vi "mainObjectivesRegistration.vi"() -> ()   [LabVIEW 2017]
uses:
  globalUtilities.vi
  globalDevices.vi
  <userlib>/Hamamatsu Video Capture/tm_getframe16_40.vi
  <vilib>/Analysis/baseanly.llb/Std Deviation and Variance.vi
  <vilib>/Analysis/NI_AALPro.lvlib
panel:
  in  "galvo N-1 2":i32
  in  "piezo M 2":i32=1
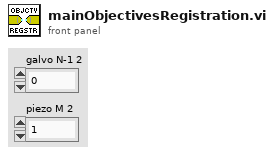
[diagram p1: front panel]
types:
  T1 = cluster{"initial amplitude":dbl, "initial center":dbl, "initial standard deviation":dbl, "offset":dbl}
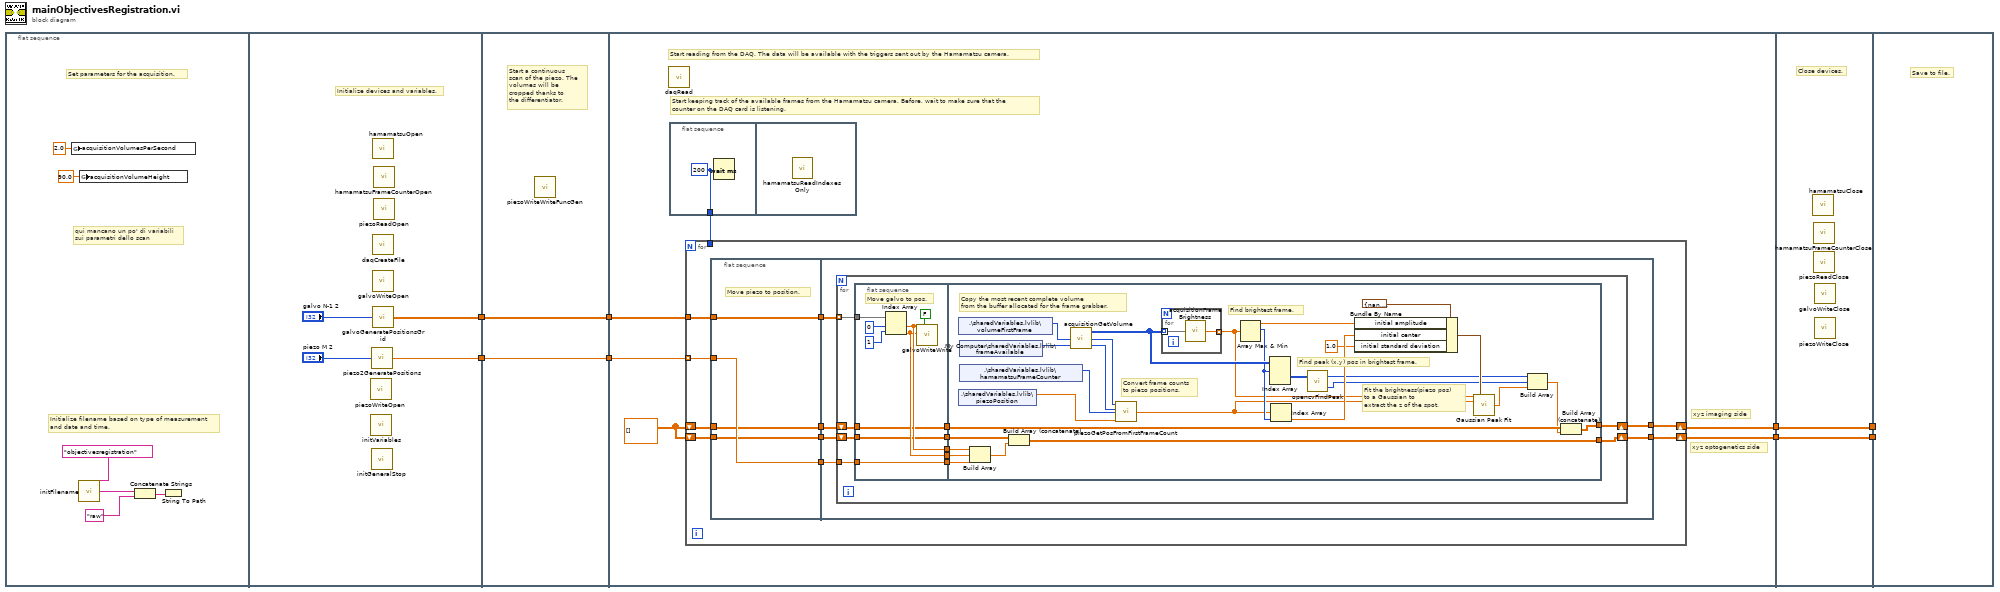
[diagram p0: block diagram]
diagram:
  n1 = flat-sequence {
    tunnel: [w16] -> w7
    tunnel: [w15] -> w5
    tunnel: [w20] -> w8
    tunnel: w7 -> [w20]
    tunnel: [w19] -> w6
    tunnel: w5 -> [w19]
    tunnel: w8 -> [w26]
    tunnel: w6 -> [w25]
    tunnel: [w23] -> w4
    tunnel: [w22] -> w3
    tunnel: w4 -> [w99]
    tunnel: w3 -> [w98]
    tunnel: [w99] -> w2
    tunnel: [w98] -> w1
    tunnel: w2 -> [_]
    tunnel: w1 -> [_]
    frame #0 {
      # "Initialize filename based on type of measurement\nand date and time."
      # "qui mancano un po' di variabili\nsui parametri dello scan"
      # "Set parameters for the acquisition."
      n2 = global write "globalUtilities.vi" "acquisitionVolumesPerSecond"(2.0 ("acquisitionVolumesPerSecond")) -> ()
      n3 = call "initFilename.vi"("Experiment type"="objectivesregistration") -> ("folder name"=w9:string)  [unwired: 1 in]
      n4 = global write "globalUtilities.vi" "acquisitionVolumeHeight"(90.0 ("acquisitionVolumeHeight")) -> ()
      n5 = Concatenate Strings(w9, "raw") -> (w10:string)
      n6 = String To Path(string=w10) -> ()  [unwired: 1 out]
    }
    frame #1 {
      # "Initialize devices and variables."
      n7 = call "piezoWriteOpen.vi"() -> ()  [unwired: 2 in]
      n8 = call "initVariables.vi"() -> ()  [unwired: 12 in]
      n9 = call "piezo2GeneratePositions.vi"("M"="piezo M 2") -> ("positions (z)"=w15:dbl[])
      n10 = call "initGeneralStop.vi"() -> ()  [unwired: 1 in]
      n11 = call "hamamatsuOpen.vi"() -> ()  [unwired: 4 out]
      n12 = call "daqCreateFile.vi"() -> ()  [unwired: 12 in]
      n13 = call "galvoWriteOpen.vi"() -> ()  [unwired: 12 in]
      n14 = call "galvoGeneratePositionsGrid.vi"("N-1"="galvo N-1 2") -> ("grid"=w16:dbl[][])
      n15 = call "hamamatsuFrameCounterOpen.vi"() -> ()  [unwired: 12 in]
      n16 = call "piezoReadOpen.vi"() -> ()  [unwired: 6 in]
    }
    frame #2 {
      # "Start a continuous\nscan of the piezo. The \nvolumes will be\ncropped thanks to\nthe differentiator."
      n17 = call "piezoWriteWriteFuncGen.vi"() -> ()  [unwired: 12 in]
    }
    frame #3 {
      w24 = dbl[][] []
      # "Start keeping track of the available frames from the Hamamatsu camera. Before, wait to make sure that the\ncounter on the DAQ card is listening."
      # "Start reading from the DAQ. The data will be available with the triggers sent out by the Hamamatsu camera."
      # "xyz optogenetics side"
      # "xyz imaging side"
      n18 = call "daqRead.vi"() -> ()  [unwired: 3 in]
      n19 = flat-sequence {
        tunnel: [w97] -> w21
        frame #0 {
          w97 = u32 200 ("milliseconds to wait")
          n20 = Wait (ms)(milliseconds to wait=w97) -> ()  [unwired: 1 out]
        }
        frame #1 {
          n21 = call "hamamatsuReadIndexesOnly.vi"() -> ()  [unwired: 12 in]
        }
      }
      n22 = for {
        tunnel: w26 -> [w34]
        tunnel: w25 -> [w36] mode=indexing
        shift-right: [w29] -> w23
        shift-left: w24 -> [w32]
        shift-right: [w27] -> w22
        shift-left: w24 -> [w30]
        tunnel: w21 -> [_]
        n23 = flat-sequence {
          tunnel: w36 -> [w39]
          tunnel: [w40] -> w35
          tunnel: w34 -> [w40]
          tunnel: [w39] -> w33
          tunnel: w32 -> [w38]
          tunnel: [w38] -> w31
          tunnel: w30 -> [w37]
          tunnel: [w37] -> w28
          tunnel: w35 -> [w46]
          tunnel: w33 -> [w45]
          tunnel: w31 -> [w44]
          tunnel: [w43] -> w29
          tunnel: w28 -> [w42]
          tunnel: [w41] -> w27
          frame #0 {
            # "Move piezo to position."
          }
          frame #1 {
            n24 = for {
              tunnel: w46 -> [w57] mode=indexing
              tunnel: w45 -> [w53]
              shift-right: [w50] -> w43
              shift-left: w44 -> [w51]
              shift-right: [w47] -> w41
              shift-left: w42 -> [w48]
              n25 = flat-sequence {
                tunnel: w57 -> [w64]
                tunnel: [w62] -> w56
                tunnel: [w61] -> w55
                tunnel: [w60] -> w54
                tunnel: w53 -> [w60]
                tunnel: [w59] -> w52
                tunnel: w51 -> [w59]
                tunnel: [w58] -> w49
                tunnel: w48 -> [w58]
                tunnel: w56 -> [w72]
                tunnel: w55 -> [w71]
                tunnel: w54 -> [w70]
                tunnel: w52 -> [w75]
                tunnel: [w73] -> w50
                tunnel: w49 -> [w69]
                tunnel: [w67] -> w47
                frame #0 {
                  # "Move galvo to pos."
                  n26 = Index Array(array=w64, index #1=0 ("index"), index #2=1 ("index")) -> (element #1=w62:dbl, element #2=w61:dbl)
                  n27 = call "galvoWriteWrite.vi"("X"=w62, "Y"=w61, "fractional units (T)"=FALSE) -> ()  [unwired: 3 in]
                }
                frame #1 {
                  # "Find peak (x,y) pos in brightest frame."
                  # "Find brightest frame."
                  # "Convert frame counts\nto piezo positions."
                  # "Copy the most recent complete volume\nfrom the buffer allocated for the frame grabber."
                  # "Fit the brightness(piezo pos) \nto a Gaussian to\nextract the z of the spot."
                  n28 = shared-variable ".\\sharedVariables.lvlib\\volumeFirstFrame"() -> (w94:u32[])  [unwired: 1 in, 1 out]
                  n29 = shared-variable ".\\sharedVariables.lvlib\\piezoPosition"() -> (w89:dbl[])  [unwired: 1 in, 1 out]
                  n30 = shared-variable "My Computer\\sharedVariables.lvlib\\frameAvailable"() -> (w93:i32[])  [unwired: 1 in, 1 out]
                  n31 = shared-variable ".\\sharedVariables.lvlib\\hamamatsuFrameCounter"() -> (w90:u32[])  [unwired: 1 in, 1 out]
                  n32 = Build Array(w72, w71, w70) -> (w68:dbl[])
                  n33 = Build Array (concatenate)(w69, w68) -> (w67:dbl[][])
                  n34 = call "acquisitionGetVolume.vi"("frameAvailable"=w93, "volumeFirstFrame"=w94) -> ("numberOfFrames"=w91:u32, "absoluteCountFirstFrame"=w92:u32, "volume out"=w88:u16[][][])  [unwired: 1 in]
                  n35 = call "piezoGetPosFromFirstFrameCount.vi"("piezoPosition"=w89, "hamamatsuFrameCounter"=w90, "numberOfFrames"=w91, "firstFrameCount"=w92) -> ("piezo pos out"=w81:dbl[])  [unwired: 2 in]
                  n36 = for {
                    tunnel: w88 -> [w96] mode=indexing
                    tunnel: [w95] -> w80 mode=indexing
                    n37 = call "acquisitionFrameBrightness.vi"("frame"=w96) -> ("brighness"=w95:dbl)
                  }
                  n38 = Array Max & Min(array=w80) -> (max value=w85:dbl, max index (indices)=w86:i32)  [unwired: 2 out]
                  n39 = Index Array(array=w88, index (dim 0)=w86) -> (element=w87:u16[][])  [unwired: 2 in]
                  n40 = Index Array(array=w81, index=w86) -> (element=w84:dbl)
                  n41 = call "opencvFindPeak.vi"("Image (2D)"=w87) -> ("maxLocY"=w77:i32, "maxLocX"=w78:i32)  [unwired: 1 in]
                  n42 = Bundle By Name(cluster=T1 {"initial amplitude"=nan, "initial center"=nan, "initial standard deviation"=1.0, "offset"=0.0} ("initial guess"), "initial amplitude"=w85, "initial center"=w84, "initial standard deviation"=1.0) -> (w79:T1)
                  n43 = call <vilib>:"Gaussian Peak Fit.vi"("Y"=w80, "initial guess"=w79, "X"=w81) -> ("center"=w76:dbl)  [unwired: 6 in, 6 out]
                  n44 = Build Array(w78, w77, w76) -> (w74:dbl[])
                  n45 = Build Array (concatenate)(w75, w74) -> (w73:dbl[][])
                }
              }
            }
          }
        }
      }
    }
    frame #4 {
      # "Close devices."
      n46 = call "hamamatsuClose.vi"() -> ()  [unwired: 1 out]
      n47 = call "hamamatsuFrameCounterClose.vi"() -> ()  [unwired: 12 in]
      n48 = call "piezoReadClose.vi"() -> ()  [unwired: 1 in]
      n49 = call "galvoWriteClose.vi"() -> ()  [unwired: 12 in]
      n50 = call "piezoWriteClose.vi"() -> ()  [unwired: 1 in]
    }
    frame #5 {
      # "Save to file."
    }
  }
